vi "waitForTemperature.vi"(4 "Type":enum16{"In Range", "Less", "Greater"}(ring), 6 "Channel":i32, 8 "error in (no error)":errorcluster, 9 "Tolerance (K)":dbl=0.005, 10 "Setpoint (K)":dbl, 11 "Instrument.Cryostat in":refnum<class "Instrument.Cryostat.lvclass">) -> (0 "error out":errorcluster, 3 "Instrument.Cryostat out":refnum<class "Instrument.Cryostat.lvclass">)   [LabVIEW 2019, in "Instrument.Cryostat.lvclass"]
uses:
  Instrument.Cryostat.lvclass
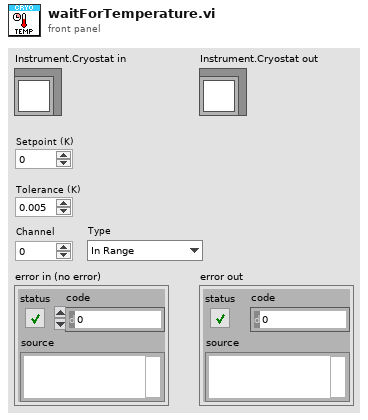
[diagram p1: front panel]
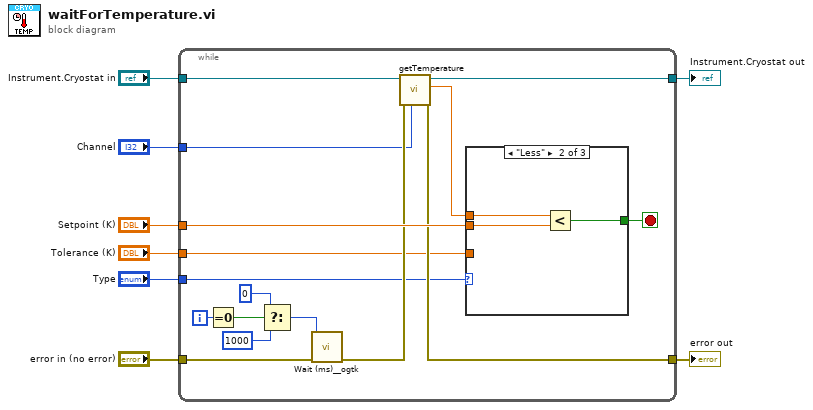
[diagram p0: block diagram]
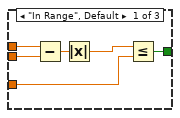
[diagram p2: hidden frame]
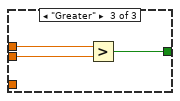
[diagram p3: hidden frame]
diagram:
  n1 = while {
    tunnel: "Setpoint (K)" -> [w24]
    tunnel: "Instrument.Cryostat in" -> [w18]
    tunnel: "error in (no error)" -> [w19]
    tunnel: [w22] -> w7
    tunnel: [w17] -> w8
    tunnel: "Channel" -> [w16]
    tunnel: "Type" -> [w15]
    tunnel: "Tolerance (K)" -> [w14]
    i -> [w12]
    stop <- w21 stop-if-true
    n2 = Equal To 0?(x=w12) -> (x = 0?=w13:bool)
    n3 = Select(t=u32 0, s=w13, f=u32 1000 ("milliseconds to wait")) -> (s? t:f=w11:u32)
    n4 = call <userlib>:"Wait (ms)__ogtk.vi"("error in (no error)"=w19, "milliseconds to wait"=w11) -> ("error out"=w23:errorcluster)  [unwired: 8 in, 1 out]
    n5 = call-dynamic "getTemperature.vi"("Channel"=w16, "error in (no error)"=w23, "Instrument.Cryostat in"=w18) -> ("error out"=w22:errorcluster, "Temperature (K)"=w20:dbl, "Instrument.Cryostat out"=w17:refnum<class "Instrument.Cryostat.lvclass">)  [unwired: 4 in, 2 out]
    n6 = case shown="\"Less\"" w15 {
      tunnel: w24 -> [w28 w33 w36]
      tunnel: [w27 w31 w34] -> w21
      tunnel: w20 -> [w26 w32 w35]
      tunnel: w14 -> [w25 _ _]
      frame "In Range", Default {
        n7 = Subtract(x=w26, y=w28) -> (x-y=w30:dbl)
        n8 = Absolute Value(x=w30) -> (abs(x)=w29:dbl)
        n9 = Less Or Equal?(x=w29, y=w25) -> (x <= y?=w27:bool)
      }
      frame "Less" {
        n10 = Less?(x=w32, y=w33) -> (x < y?=w31:bool)
      }
      frame "Greater" {
        n11 = Greater?(x=w35, y=w36) -> (0:w34:bool)
      }
    }
  }
  "Instrument.Cryostat out" <- w8
  "error out" <- w7
